vi "Read configuration.vi"(7 "force loading?":bool=TRUE, 8 "error in (no error)":errorcluster, 11 "MeritFactor in":refnum<class "MeritFactor.lvclass">) -> (0 "error out":errorcluster, 3 "MeritFactor out":refnum<class "MeritFactor.lvclass">)   [LabVIEW 2012, in "MeritFactor.lvclass"]
doc: "Reads the XML-based configuration file and populates the configuration cluster accordingly. Configuration file name is <component ID>.xml."
uses:
  MeritFactor.lvclass
  <vilib>/Distrio/Murmex/Murmex/Murmex.lvclass
  MeritFactor.lvclass/MeritFactor.ctl
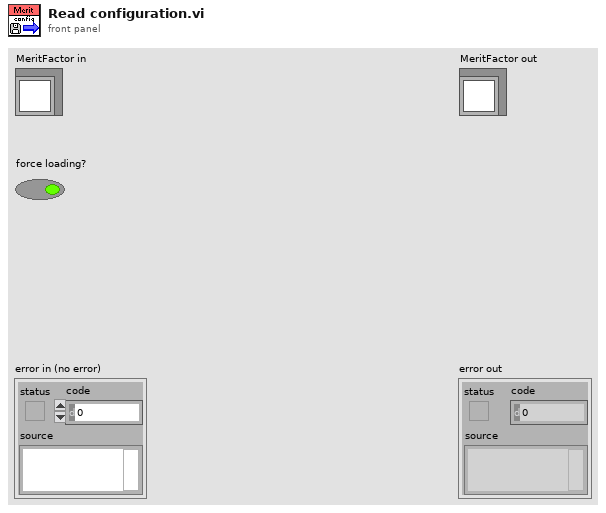
[diagram p1: front panel]
types:
  T1 = typedef "MeritFactor.lvclass/configuration cluster.ctl" = cluster{"Merit factor type":T2}
  T2 = typedef "MeritFactor.lvclass/merit factor type.ctl" = enum16{"Full frame intensity", "Brightest pixels intensity", "Contrast"}
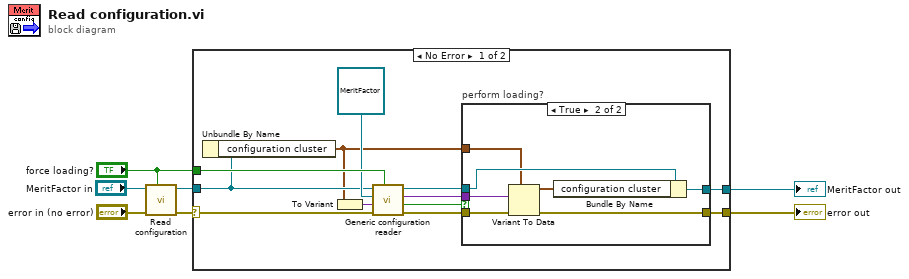
[diagram p0: block diagram]
diagram:
  n1 = call-parent "Read configuration.vi"("force loading?"="force loading?", "error in (no error)"="error in (no error)", "Murmex in"="MeritFactor in") -> ("error out"=w5:errorcluster, "Murmex out"=w4:refnum<class "MeritFactor.lvclass">)  [unwired: 7 in]
  n2 = case shown="No Error" w5 {
    selector: w5 -> [w19 w29]
    tunnel: w4 -> [w16 w30]
    tunnel: "force loading?" -> [w18 _]
    tunnel: [w9 w29] -> w2
    tunnel: [w8 w30] -> w1
    frame No Error {
      n3 = Unbundle By Name(w16) -> ("configuration cluster"=w10:T1)
      n4 = To Variant(anything=w10) -> (Variant=w15:variant)
      n5 = call <vilib>:"Generic configuration reader.vi"("force loading?"=w18, "error in (no error)"=w19, "configuration cluster variant"=w15, "inheritance level"=refnum<class "MeritFactor.lvclass"> refnum ("MeritFactor"), "Murmex in"=w16) -> ("error out"=w13:errorcluster, "loaded?"=w14:bool, "configuration data (variant)"=w12:variant, "Murmex out"=w11:refnum<class "MeritFactor.lvclass">)  [unwired: 3 in]
      n6 = case "perform loading?" shown="True" w14 {
        tunnel: w13 -> [w20 w28]
        tunnel: w12 -> [_ w27]
        tunnel: w11 -> [w21 w26]
        tunnel: [w21 w24] -> w8
        tunnel: w10 -> [_ w23]
        tunnel: [w20 w22] -> w9
        frame False {
        }
        frame True {
          n7 = Variant To Data(error in=w28, type=w23, Variant=w27) -> (data=w25:T1, error out=w22:errorcluster)
          n8 = Bundle By Name(cluster=w26, "configuration cluster"=w25) -> (w24:refnum<class "MeritFactor.lvclass">)
        }
      }
    }
    frame Error {
    }
  }
  "error out" <- w2
  "MeritFactor out" <- w1
